vi "Stream FPGA Data.vi"(9 "TDMS file base path":path, 10 "DMA Data Values":u64[](array[numeric]), 11 "tdms file in":refnum<k34>) -> (0 "error out":errorcluster, 2 "[I16] All points in correct chronological order":i16[](array[numeric]), 3 "tdms file out":refnum<k34>)   [LabVIEW 2020]
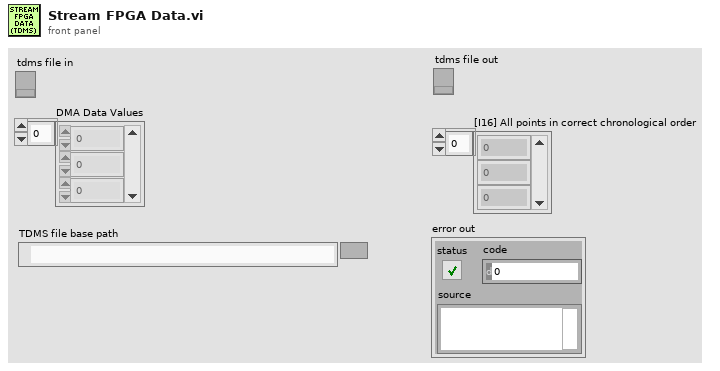
[diagram p1: front panel]
types:
  T1 = enum16{"open", "open or create", "create or replace", "create", "open (read-only)"}
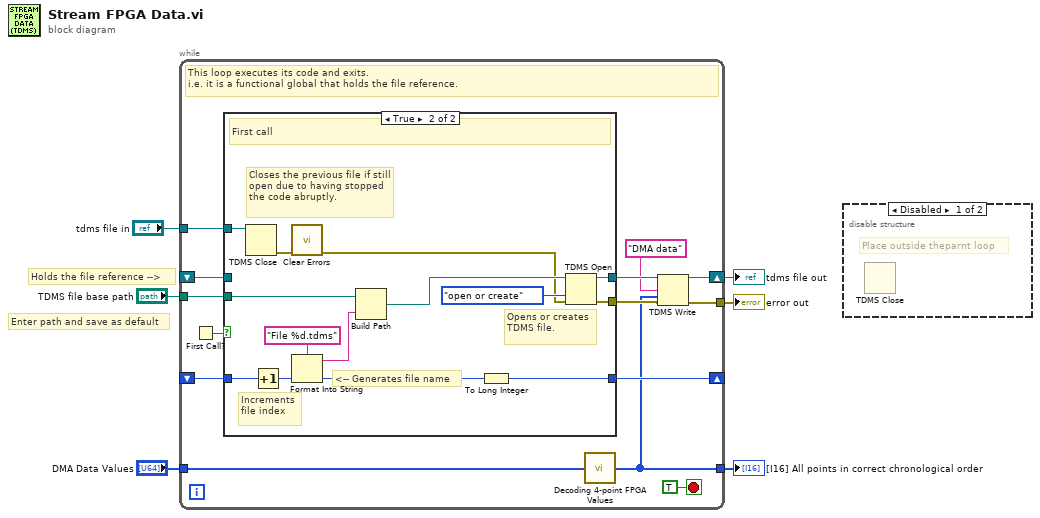
[diagram p0: block diagram]
diagram:
  # "Holds the file reference -->"
  # "Enter path and save as default"
  n1 = while {
    shift-right: [w16] -> w6
    shift-left: _ -> [w18]
    shift-right: [w13] -> _
    shift-left: _ -> [w20]
    tunnel: "TDMS file base path" -> [w14]
    tunnel: "DMA Data Values" -> [w12]
    tunnel: [w11] -> w3
    tunnel: "tdms file in" -> [w9]
    tunnel: [w8] -> w1
    stop <- TRUE stop-if-true
    # "This loop executes its code and exits.\ni.e. it is a functional global that holds the file reference."
    n2 = First Call?() -> (First Call?: T/F=w19:bool)
    n3 = case shown="True" w19 {
      tunnel: w20 -> [w21 w31]
      tunnel: [w22 w34] -> w15
      tunnel: w18 -> [w22 _]
      tunnel: w14 -> [_ w33]
      tunnel: [w21 w23] -> w13
      tunnel: [_ w27] -> w10
      tunnel: w9 -> [_ w25]
      frame False {
        # "Consecutive calls"
      }
      frame True {
        # "Opens or creates TDMS file."
        # "<-- Generates file name"
        # "Increments file index"
        # "Closes the previous file if still open due to having stopped the code abruptly."
        # "First call"
        n4 = TDMS Close(11:w25) -> (0:w26:errorcluster)  [unwired: 1 in, 1 out]
        n5 = Increment(x=w31) -> (x+1=w28:i32)
        n6 = call <vilib>:"Clear Errors.vi"("error in (no error)"=w26) -> ("error out"=w24:errorcluster)  [unwired: 5 in, 1 out]
        n7 = Format Into String(format string="File %d.tdms", w28) -> (resulting string=w29:string)  [unwired: 2 in, 1 out]
        n8 = Build Path(base path=w33, name or relative path=w29) -> (appended path=w32:path)
        n9 = To Long Integer(number=w28) -> (32bit integer=w23:i32)
        n10 = TDMS Open(8:w24, 10:T1."open or create" ("operation (0:open)"), 11:w32) -> (0:w27:errorcluster, 3:w34:refnum<k34>)  [unwired: 4 in]
      }
    }
    n11 = call "Decoding 4-point FPGA Values.vi"("DMA Data"=w12) -> ("[I16] All points in correct chronological order"=w8:i16[])
    n12 = TDMS Write(0:w15, 7:"DMA data", 9:w8, 11:w10) -> (4:w16:refnum<k34>, 15:w11:errorcluster)  [unwired: 2 in, 2 out]
  }
  "tdms file out" <- w6
  "error out" <- w3
  "[I16] All points in correct chronological order" <- w1
  n13 = disable-structure "Diagram Disable Structure" shown="Disabled" {
    frame Disabled {
      # "Place outside theparnt loop"
      n14 = TDMS Close() -> ()  [unwired: 2 in, 2 out]
    }
    frame Enabled {
    }
  }
